vi "Error.vi"(8 "error in (no error)":errorcluster, 11 "main queue":refnum<queue>) -> (0 "error out":errorcluster)   [LabVIEW 2025, in "Config Tool.lvlib"]
doc: "Enqueues the error as a message so it can be hanlde in the error caseCopyright 2017 National Instruments Corporation\n\nLicensed under the Apache License, Version 2.0 (the \"License\"); you may not use this file except in compliance with the License. You may obtain a copy of the License at http://www.apache.org/licenses/LICENSE-2.0\nUnless required by applicable law or agreed to in writing, software distributed under the License is distributed on an \"AS IS\" BASIS, WITHOUT WARRANTIES OR CONDITIONS OF ANY KIND, either express or implied. See the License for the specific language governing permissions and limitations under the License."
uses:
  Config Tool.lvlib
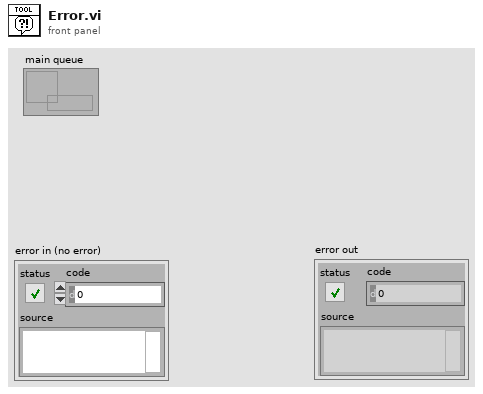
[diagram p1: front panel]
types:
  T1 = cluster{"message name":string, "data string":string}
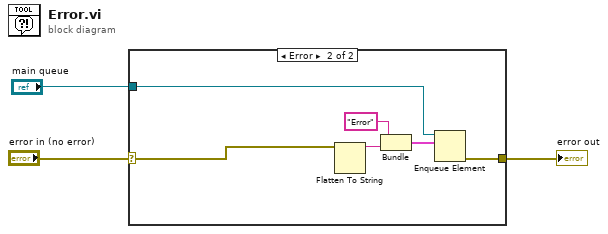
[diagram p0: block diagram]
diagram:
  n1 = case shown="Error" "error in (no error)" {
    selector: "error in (no error)" -> [w4 w6]
    tunnel: [w4 w10] -> w3
    tunnel: "main queue" -> [_ w9]
    frame No Error {
    }
    frame Error {
      n2 = Flatten To String(anything=w6) -> (data string=w5:string)  [unwired: 3 in, 2 out]
      n3 = Bundle("message name"="Error", "data string"=w5) -> (w7:T1)  [unwired: 1 in]
      n4 = Enqueue Element(queue=w9, element=w7) -> (error out=w10:errorcluster)  [unwired: 2 in, 2 out]
    }
  }
  "error out" <- w3
